vi "get Port Name.vi"(11 "port_num":i32) -> (3 "function return":string)   [LabVIEW 2021, in "dxl_x86_c.lvlib"]
doc: "WINDECLSPEC char *getPortName (int port_num);"
uses:
  dxl_x86_c.lvlib
  dxl_x86_c.dll
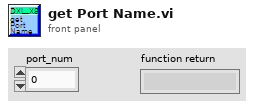
[diagram p1: front panel]
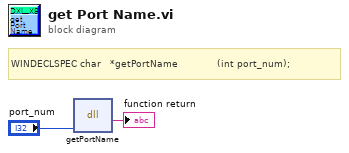
[diagram p0: block diagram]
diagram:
  # "WINDECLSPEC char   *getPortName             (int port_num);"
  n1 = dll-call lib="C:/Users/ashek/Desktop/ashekim/ws/DynamixelSDK/labview/labview/dxl_x86_c.*" fn="getPortName"("port_num"="port_num") -> (→"function return":string)  [unwired: 4 in, 2 out]
